vi "Buffer Load L.vi"(8 "Error In":errorcluster, 11 "On/Off":bool) -> (0 "Error Out":errorcluster)   [LabVIEW 2019, in "sbRIO9623.lvlib"]
uses:
  sbRIO9623.lvlib
  Queues/Queues.lvlib
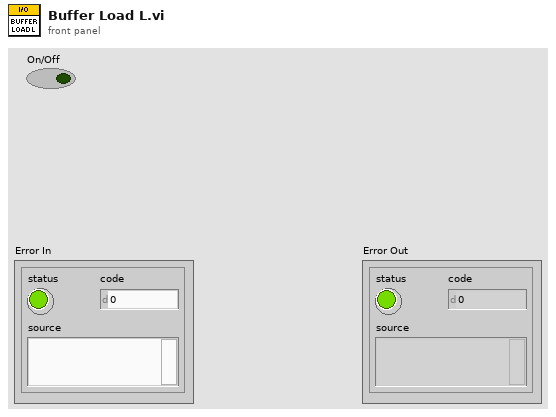
[diagram p1: front panel]
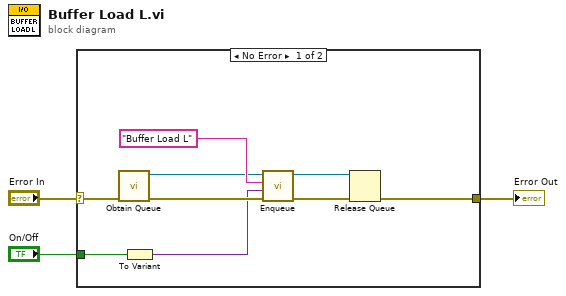
[diagram p0: block diagram]
diagram:
  n1 = case shown="No Error" "Error In" {
    selector: "Error In" -> [w8 w13]
    tunnel: [w9 w13] -> w3
    tunnel: "On/Off" -> [w5 _]
    frame No Error {
      n2 = call "Obtain Queue.vi"("Error In"=w8) -> ("Error Out"=w7:errorcluster, "Queue out"=w6:refnum<queue>)  [unwired: 9 in]
      n3 = To Variant(anything=w5) -> (Variant=w4:variant)
      n4 = call "Enqueue.vi"("Error In"=w7, "Data"=w4, "State"="Buffer Load L", "Queue in"=w6) -> ("Error Out"=w11:errorcluster, "Queue out"=w10:refnum<queue>)  [unwired: 6 in]
      n5 = Release Queue(queue=w10, error in (no error)=w11) -> (error out=w9:errorcluster)  [unwired: 1 in, 2 out]
    }
    frame Error {
    }
  }
  "Error Out" <- w3
